vi "dat_voltage_current.vi"() -> (14 "avb_p1_v":fxp<+/-,24,5>, 15 "avb_p2_v":fxp<+/-,24,5>, 16 "avb_r_v":fxp<+/-,24,5>, 17 "avb_p1_c":fxp<+/-,24,5>, 18 "avb_p2_c":fxp<+/-,24,5>, 19 "avb_r_c":fxp<+/-,24,5>)   [LabVIEW 2018]
uses:
  <vilib>/rvi/Emulation/niFpgaEmulationIsFPGAContextNoSignature.vi
  <vilib>/rvi/DataTransferAndStorage/Container/Common/niFpgaContainerGetUniqueNameForEmu.vi
  <vilib>/rvi/Memory/Memory_Emulation/niFpgaMemoryEmulationCacheClearOnFirstRun.vi
  <vilib>/rvi/Memory/Memory_Emulation/nirvimemoryEmulationManagerCache_MakeExclusive.vi
  <vilib>/rvi/Memory/Memory_Emulation/niFpgaMemoryEmulationValidateCache.vi
  <vilib>/rvi/Memory/Memory_Emulation/nirvimemoryEmulationManagerCache_InsertValue.vi
  <vilib>/Utility/error.llb/Clear Errors.vi
  <vilib>/rvi/Memory/Memory_Emulation/nirvimemoryEmulationManagerCache_ReleaseExclusive.vi
  <vilib>/rvi/Memory/Memory_Emulation/nirvimemoryEmulationManagerCache_GetValue.vi
  <vilib>/rvi/Memory/Memory_Emulation/nirvimemoryEmulationManagerCache_SetValue.vi
  <vilib>/rvi/Emulation/niFpgaProcessEmulError.vi
  <vilib>/rvi/Emulation/niFpgaSctlEmulationGetInTimedLoop.vi
  <vilib>/rvi/DataTransferAndStorage/Container/XNode/niFpgaContainer.xnode
  <vilib>/rvi/DataTransferAndStorage/Register/Emulation/niFpgaRegisterEmulation.vi
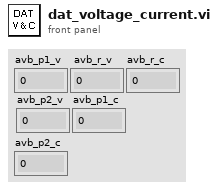
[diagram p1: front panel]
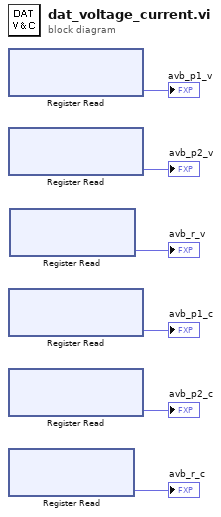
[diagram p0: block diagram]
diagram:
  n1 = xnode "Register Read"() -> ("Data"=→"avb_p1_v":fxp<+/-,24,5>)  [unwired: 1 in, 1 out]
  n2 = xnode "Register Read"() -> ("Data"=→"avb_p2_v":fxp<+/-,24,5>)  [unwired: 1 in, 1 out]
  n3 = xnode "Register Read"() -> ("Data"=→"avb_p1_c":fxp<+/-,24,5>)  [unwired: 1 in, 1 out]
  n4 = xnode "Register Read"() -> ("Data"=→"avb_p2_c":fxp<+/-,24,5>)  [unwired: 1 in, 1 out]
  n5 = xnode "Register Read"() -> ("Data"=→"avb_r_c":fxp<+/-,24,5>)  [unwired: 1 in, 1 out]
  n6 = xnode "Register Read"() -> ("Data"=→"avb_r_v":fxp<+/-,24,5>)  [unwired: 1 in, 1 out]
